vi "U8Array-to-U64Array.vi"(11 "Array in":u8[](array[numeric]) format="%.0x") -> (3 "Array out":u64[](array[numeric]) format="%.0x")   [LabVIEW 2017]
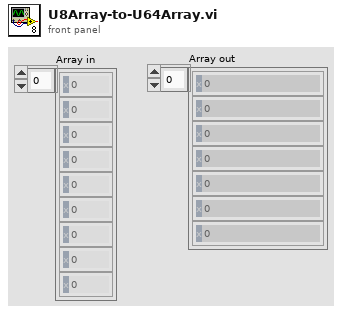
[diagram p1: front panel]
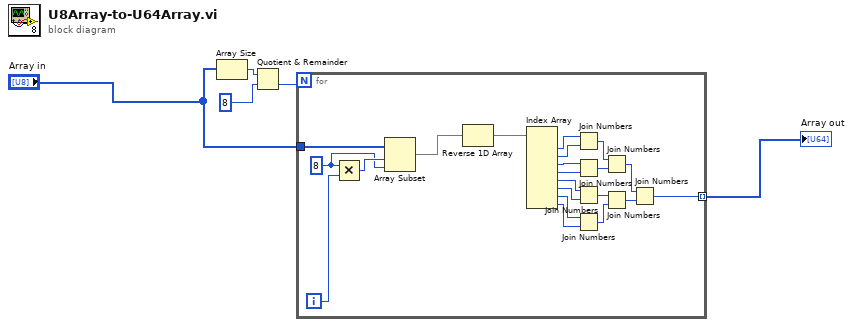
[diagram p0: block diagram]
diagram:
  n1 = Array Size(array="Array in") -> (size(s)=w2:i32)
  n2 = Quotient & Remainder(x=w2, y=8) -> (floor(x/y)=w1:i32)  [unwired: 1 out]
  n3 = for {
    N: w1 -> [_]
    tunnel: "Array in" -> [w11]
    tunnel: [w6] -> w5 mode=indexing
    i -> [w9]
    w8 = 8 ("x")
    n4 = Multiply(x=w8, y=w9) -> (x*y=w10:i32)
    n5 = Array Subset(array=w11, index=w10, length=w8) -> (w7:u8[])
    n6 = Reverse 1D Array(array=w7) -> (reversed array=w12:u8[])
    n7 = Index Array(array=w12) -> (element #1=w20:u8, element #2=w19:u8, element #3=w18:u8, element #4=w17:u8, element #5=w15:u8, element #6=w16:u8, element #7=w14:u8, element #8=w13:u8)  [unwired: 8 in]
    n8 = Join Numbers(hi=w20, lo=w19) -> ((hi.lo)=w24:u16)
    n9 = Join Numbers(hi=w18, lo=w17) -> ((hi.lo)=w23:u16)
    n10 = Join Numbers(hi=w15, lo=w16) -> ((hi.lo)=w22:u16)
    n11 = Join Numbers(hi=w14, lo=w13) -> ((hi.lo)=w21:u16)
    n12 = Join Numbers(hi=w24, lo=w23) -> ((hi.lo)=w25:u32)
    n13 = Join Numbers(hi=w22, lo=w21) -> ((hi.lo)=w26:u32)
    n14 = Join Numbers(hi=w25, lo=w26) -> ((hi.lo)=w6:u64)
  }
  "Array out" <- w5
